vi "Time Manager.vi"(11 "Reset?":bool) -> (3 "Elapsed Time":u32)   [LabVIEW 2015]
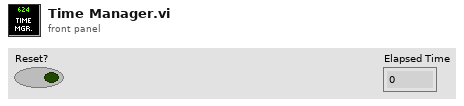
[diagram p1: front panel]
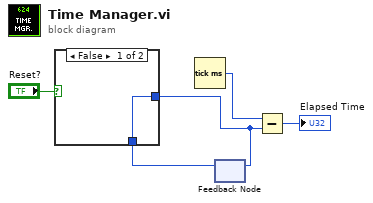
[diagram p0: block diagram]
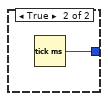
[diagram p2: hidden frame]
diagram:
  n1 = Tick Count (ms)() -> (millisecond timer value=w4:u32)
  n2 = feedback #1() -> (w2:u32)  [unwired: 1 in]
  n3 = case shown="False" "Reset?" {
    tunnel: [w6 w7] -> w3
    tunnel: w2 -> [w6 _]
    frame False {
    }
    frame True {
      n4 = Tick Count (ms)() -> (millisecond timer value=w7:u32)
    }
  }
  n5 = feedback-in #1(w3) -> ()
  n6 = Subtract(x=w4, y=w3) -> (x-y=→"Elapsed Time":u32)
